vi "stage_setup.vi"(8 "error_in":errorcluster, 9 "stage-select":T1(ring), 10 "serial-numbers":string[](array[string]), 11 ".NET Refnum in":refnum<k24>) -> (0 "error out":errorcluster, 2 "Device":refnum<k24>, 3 ".NET Refnum out":refnum<k24>)   [LabVIEW 2024]
uses:
  O:/DSG/Tyler/EIC/DIRC/daq/automated/Thorlabs.MotionControl.Controls.dll
  Thorlabs.MotionControl.Controls.dll
  O:/DSG/Tyler/EIC/DIRC/daq/automated/Thorlabs.MotionControl.IntegratedStepperMotorsCLI.dll
  Thorlabs.MotionControl.IntegratedStepperMotorsCLI.dll
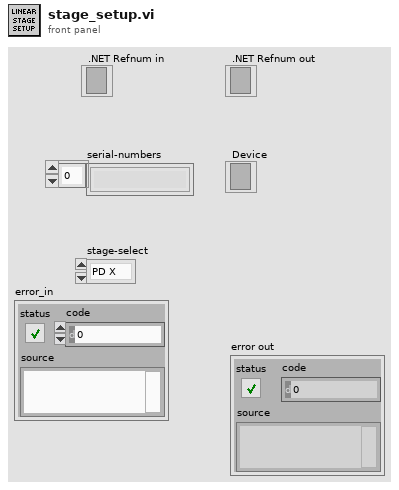
[diagram p1: front panel]
types:
  T1 = enum16{"PD X", "PD Y", "Bar X", "Bar Y", "Rotary"}
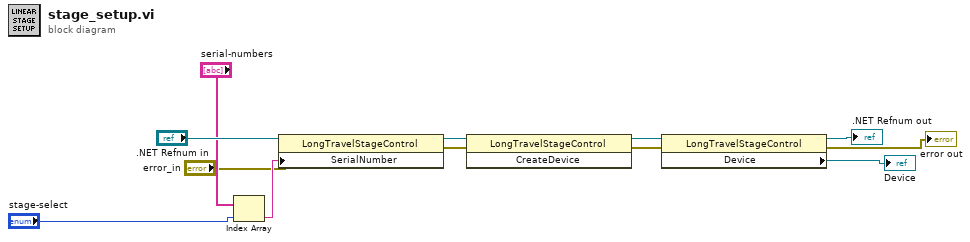
[diagram p0: block diagram]
diagram:
  n1 = Index Array(array="serial-numbers", index="stage-select") -> (element=w3:string)
  n2 = property class="LongTravelStageControl"(reference=".NET Refnum in", error in="error_in", "SerialNumber"=w3) -> (reference out=w5:refnum<k24>, error out=w6:errorcluster)
  n3 = invoke class="LongTravelStageControl" method="CreateDevice"(reference=w5, error in=w6) -> (reference out=w8:refnum<k24>, error out=w9:errorcluster)  [unwired: 1 in, 1 out]
  n4 = property class="LongTravelStageControl"(reference=w8, error in=w9) -> (reference out=→".NET Refnum out":refnum<k24>, error out=→"error out":errorcluster, "Device"=→"Device":refnum<k24>)
